vi "Queue Exists.vi"(11 "Remote VI Queue in":refnum<queue>) -> (2 "Queue Exists":bool, 3 "Remote VI Queue out":refnum<queue>)   [LabVIEW 2020, in "Dynamic Reentrant.lvlib"]
uses:
  <userlib>/DynamicReentrant/Dynamic Reentrant.lvlib
  <userlib>/DynamicReentrant/src/Type Defs/Message.ctl
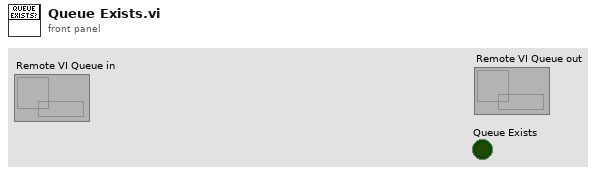
[diagram p1: front panel]
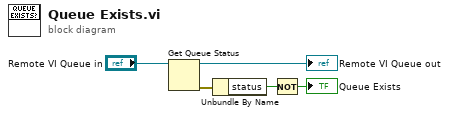
[diagram p0: block diagram]
diagram:
  n1 = Get Queue Status(queue="Remote VI Queue in") -> (queue out=→"Remote VI Queue out":refnum<queue>, error out=w3:errorcluster)  [unwired: 2 in, 6 out]
  n2 = Unbundle By Name(w3) -> ("status"=w2:bool)
  n3 = Not(x=w2) -> (.not. x?=→"Queue Exists":bool)
